vi "3-2-2 gen random data.vi"() -> (3 "output cluster":T1)   [LabVIEW 2020]
uses:
  <vilib>/numeric/Random Number (Range) DBL.vi
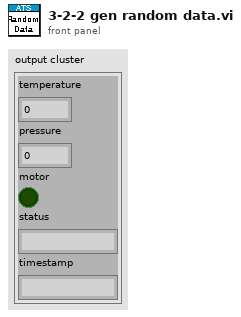
[diagram p1: front panel]
types:
  T1 = cluster{"temperature":dbl, "pressure":dbl, "motor":bool, "status":string, "timestamp":string}
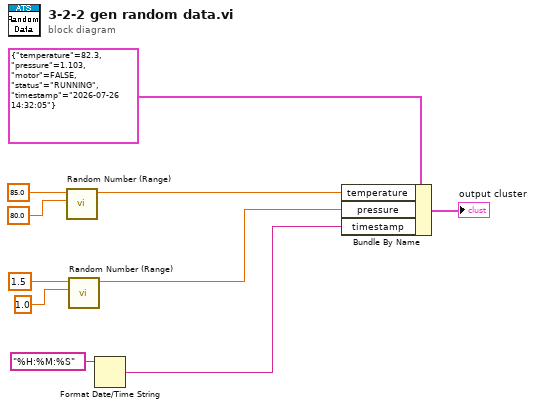
[diagram p0: block diagram]
diagram:
  n1 = call-poly <vilib>:"Random Number (Range).vi"("lower bound (0)"=80.0 ("upper bound (100)"), "upper bound (100)"=85.0) -> ("number"=w6:dbl)  [unwired: 9 in]
  n2 = call-poly <vilib>:"Random Number (Range).vi"("lower bound (0)"=1.0 ("upper bound (100)"), "upper bound (100)"=1.5) -> ("number"=w3:dbl)  [unwired: 9 in]
  n3 = Format Date/Time String(time format string (%c)="%H:%M:%S") -> (date/time string=w2:string)  [unwired: 2 in]
  n4 = Bundle By Name(cluster=T1 {"temperature"=82.3, "pressure"=1.103, "motor"=FALSE, "status"="RUNNING", "timestamp"="2026-07-26 14:32:05"} ("sensor_data"), "temperature"=w6, "pressure"=w3, "timestamp"=w2) -> (→"output cluster":T1)
